vi "Configure Crop.vi"(8 "error in (no error)":errorcluster, 9 "Codec":string, 10 "Video file path":path, 11 "Frame Grabber Data In":T1={"Camera Session"="", "Frame"=refnum, "AVI Refnum"=refnum, "Codecs"=[], "Frame number"=0, "Tracking File Refnum"=refnum, "Tick Count"=0, "Probe Object"=refnum, "Playback Probe Data"=[], "Rigid Body"={"Position"={"x (mm)"=0.0, "y (mm)"=0.0, "z (mm)"=0.0}, "Orientation"={"Pitch (rad)"=0.0, "Yaw (rad)"=0.0, "Roll (rad)"=0.0}, "Quaternion"={"qx"=0.0, "qy"=0.0, "qz"=0.0, "qw"=0.0}, "Tracked?"=FALSE}, "Total no frames playback"=0, "Video FPS"=0.0, "Camera connected?"=FALSE, "Scene"=refnum, "Cropped Frame"=refnum, "Tracker FPS"=0.0, "Crop ROI"=[], "Presentation Values"=[], "Elapsed time (ms)"=0, "Camera frames playback"=0, "Refnums"={"Live Refnum"=refnum, "Record Refnum"=refnum, "Recording Settings Refnum"=refnum, "Playback Refnum"=refnum, "Frame Slider Refnum"=refnum, "Pause Refnum"=refnum, "Home Refnum"=refnum, "Crop Refnum"=refnum, "Clear Crop Refnum"=refnum, "stop refnum"=refnum, "Playback Rate Refnum"=refnum, "Operator Settings Refnums"=refnum, "Presentation Refnum"=refnum, "Gestation Refnum"=refnum, "Connection Settings Refnum"=refnum, "Crop Time Frame Slider Refnum"=refnum}, "Dimensions"={"Probe Dimensions"={"Probe Width"=0.0, "Probe Depth"=1.0, "Probe Height"=0.0}, "Room Dimensions"={"Room Width"=0.0, "Room Depth"=0.0, "Room Height"=0.0}}, "Playback Data As Strings"=[], "Cropped Tracking File Refnum"=refnum, "Cropped AVI Refnum"=refnum, "Header"=[]}) -> (0 "error out":errorcluster, 2 "Saving?":bool, 3 "Frame Grabber Data Out":T1={"Camera Session"="", "Frame"=refnum, "AVI Refnum"=refnum, "Codecs"=[], "Frame number"=0, "Tracking File Refnum"=refnum, "Tick Count"=0, "Probe Object"=refnum, "Playback Probe Data"=[], "Rigid Body"={"Position"={"x (mm)"=0.0, "y (mm)"=0.0, "z (mm)"=0.0}, "Orientation"={"Pitch (rad)"=0.0, "Yaw (rad)"=0.0, "Roll (rad)"=0.0}, "Quaternion"={"qx"=0.0, "qy"=0.0, "qz"=0.0, "qw"=0.0}, "Tracked?"=FALSE}, "Total no frames playback"=0, "Video FPS"=0.0, "Camera connected?"=FALSE, "Scene"=refnum, "Cropped Frame"=refnum, "Tracker FPS"=0.0, "Crop ROI"=[], "Presentation Values"=[], "Elapsed time (ms)"=0, "Camera frames playback"=0, "Refnums"={"Live Refnum"=refnum, "Record Refnum"=refnum, "Recording Settings Refnum"=refnum, "Playback Refnum"=refnum, "Frame Slider Refnum"=refnum, "Pause Refnum"=refnum, "Home Refnum"=refnum, "Crop Refnum"=refnum, "Clear Crop Refnum"=refnum, "stop refnum"=refnum, "Playback Rate Refnum"=refnum, "Operator Settings Refnums"=refnum, "Presentation Refnum"=refnum, "Gestation Refnum"=refnum, "Connection Settings Refnum"=refnum, "Crop Time Frame Slider Refnum"=refnum}, "Dimensions"={"Probe Dimensions"={"Probe Width"=0.0, "Probe Depth"=1.0, "Probe Height"=0.0}, "Room Dimensions"={"Room Width"=0.0, "Room Depth"=0.0, "Room Height"=0.0}}, "Playback Data As Strings"=[], "Cropped Tracking File Refnum"=refnum, "Cropped AVI Refnum"=refnum, "Header"=[]})   [LabVIEW 2017]
uses:
  Controls/Frame Grabber Data.ctl
  <vilib>/userdefined/High Color/IMAQdx.ctl
  <vilib>/vision/Image Controls.llb/IMAQ Image.ctl
  <vilib>/vision/Avi.llb/IMAQ AVI2 Refnum.ctl
  Controls/Rigid Body Info.ctl
  Controls/Position.ctl
  Controls/Orientation.ctl
  Controls/Refnums.ctl
  Controls/Recording Settings.ctl
  Controls/Operator Settings.ctl
  Controls/Operator.ctl
  Controls/Dimensions.ctl
  Controls/Room Dimensions.ctl
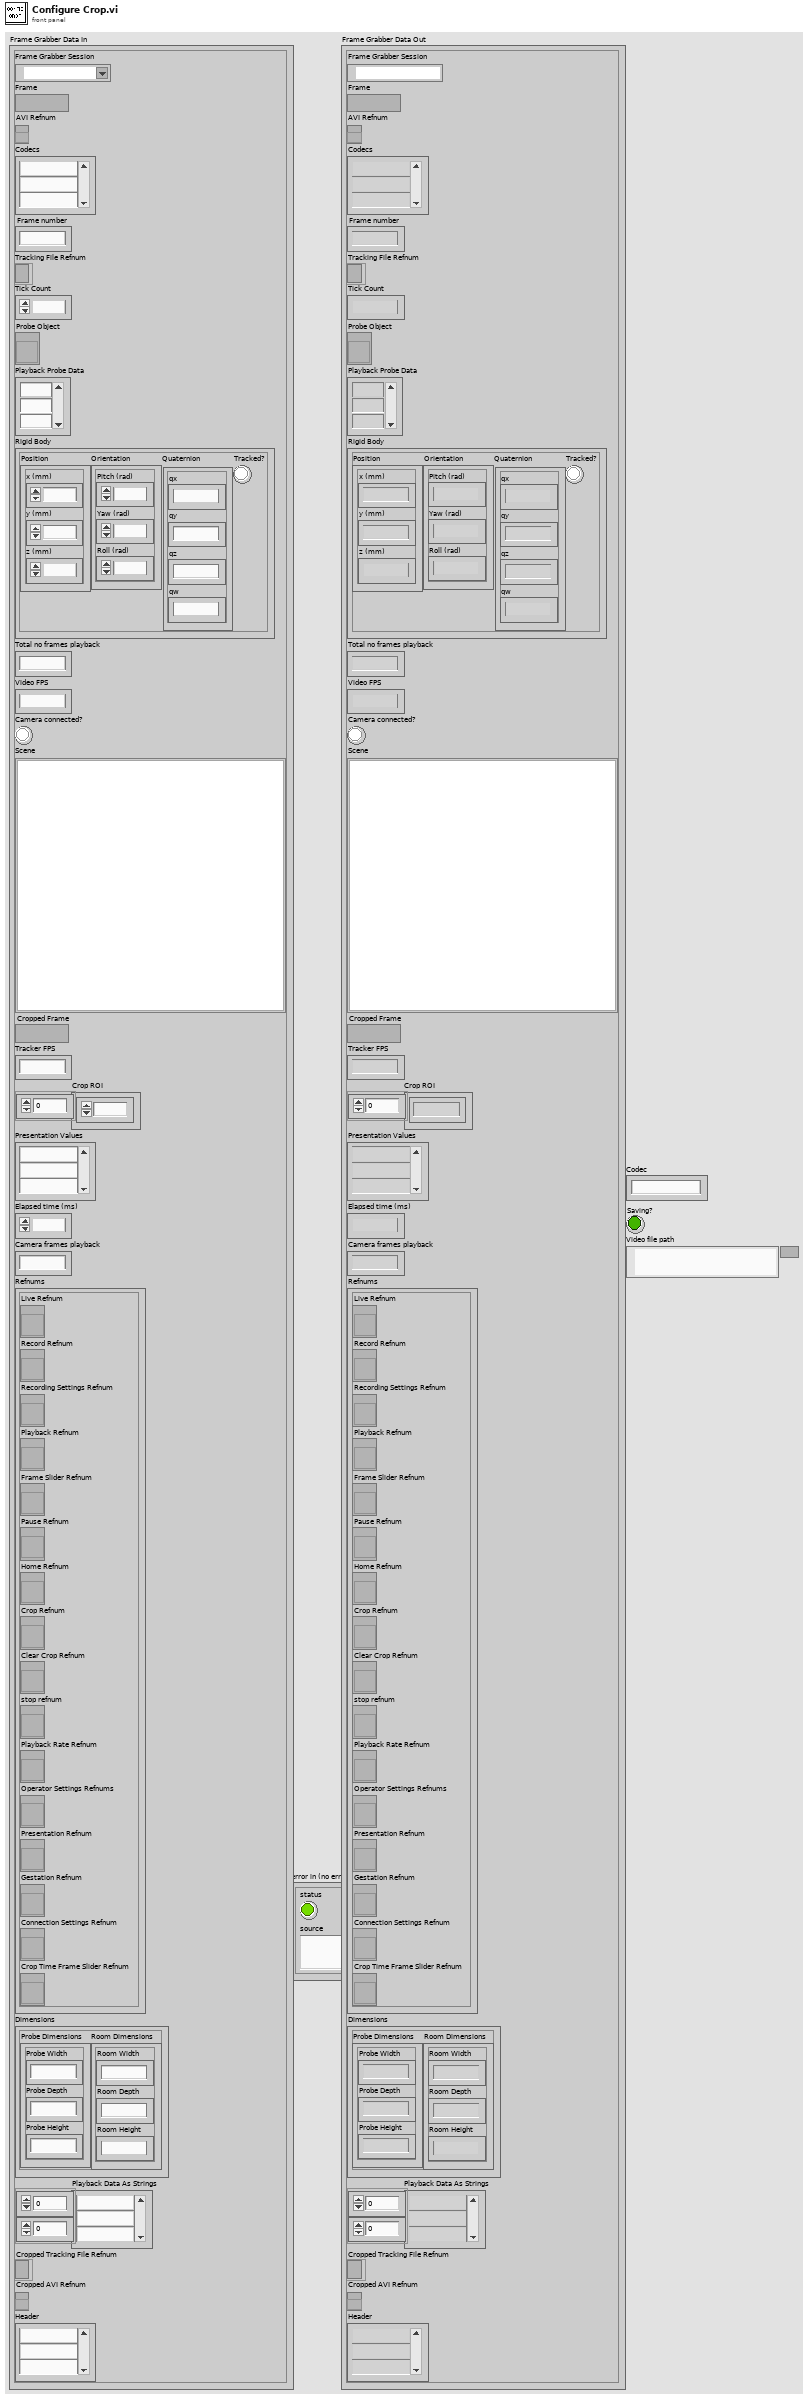
[diagram p1: front panel]
types:
  T1 = typedef "Frame Grabber Data.ctl" = cluster{"Camera Session":T2, "Frame":T3, "AVI Refnum":T4, "Codecs":string[], "Frame number":u32, "Tracking File Refnum":refnum<file>, "Tick Count":u32, "Probe Object":refnum<vi>, "Playback Probe Data":dbl[][], "Rigid Body":T5, "Total no frames playback":i32, "Video FPS":dbl, "Camera connected?":bool, "Scene":refnum<vi>, "Cropped Frame":T3, "Tracker FPS":dbl, "Crop ROI":i32[], "Presentation Values":string[], "Elapsed time (ms)":u32, "Camera frames playback":u32, "Refnums":T8, "Dimensions":T9, "Playback Data As Strings":string[][], "Cropped Tracking File Refnum":refnum<file>, "Cropped AVI Refnum":T4, "Header":string[]}
  T2 = typedef "IMAQdx.ctl" = refnum<k21>
  T3 = typedef "IMAQ Image.ctl" = refnum<image>
  T4 = typedef "IMAQ AVI2 Refnum.ctl" = refnum<k20>
  T5 = typedef "Rigid Body Info.ctl" = cluster{"Position":T6, "Orientation":T7, "Quaternion":cluster{"qx":sgl, "qy":sgl, "qz":sgl, "qw":sgl}, "Tracked?":bool}
  T6 = typedef "Position.ctl" = cluster{"x (mm)":sgl, "y (mm)":sgl, "z (mm)":sgl}
  T7 = typedef "Orientation.ctl" = cluster{"Pitch (rad)":sgl, "Yaw (rad)":sgl, "Roll (rad)":sgl}
  T8 = typedef "Refnums.ctl" = cluster{"Live Refnum":refnum<vi>, "Record Refnum":refnum<vi>, "Recording Settings Refnum":refnum<vi>, "Playback Refnum":refnum<vi>, "Frame Slider Refnum":refnum<vi>, "Pause Refnum":refnum<vi>, "Home Refnum":refnum<vi>, "Crop Refnum":refnum<vi>, "Clear Crop Refnum":refnum<vi>, "stop refnum":refnum<vi>, "Playback Rate Refnum":refnum<vi>, "Operator Settings Refnums":refnum<vi>, "Presentation Refnum":refnum<vi>, "Gestation Refnum":refnum<vi>, "Connection Settings Refnum":refnum<vi>, "Crop Time Frame Slider Refnum":refnum<vi>}
  T9 = typedef "Dimensions.ctl" = cluster{"Probe Dimensions":cluster{"Probe Width":sgl, "Probe Depth":sgl, "Probe Height":sgl}, "Room Dimensions":T10}
  T10 = typedef "Room Dimensions.ctl" = cluster{"Room Width":dbl, "Room Depth":dbl, "Room Height":dbl}
  T11 = enum16{"open", "replace", "create", "open or create", "replace or create", "replace or create with confirmation"}
  T12 = cluster{"Width":u32, "Height":u32, "Frames Per Second":u32, "Codec":string, "Has Data":bool}
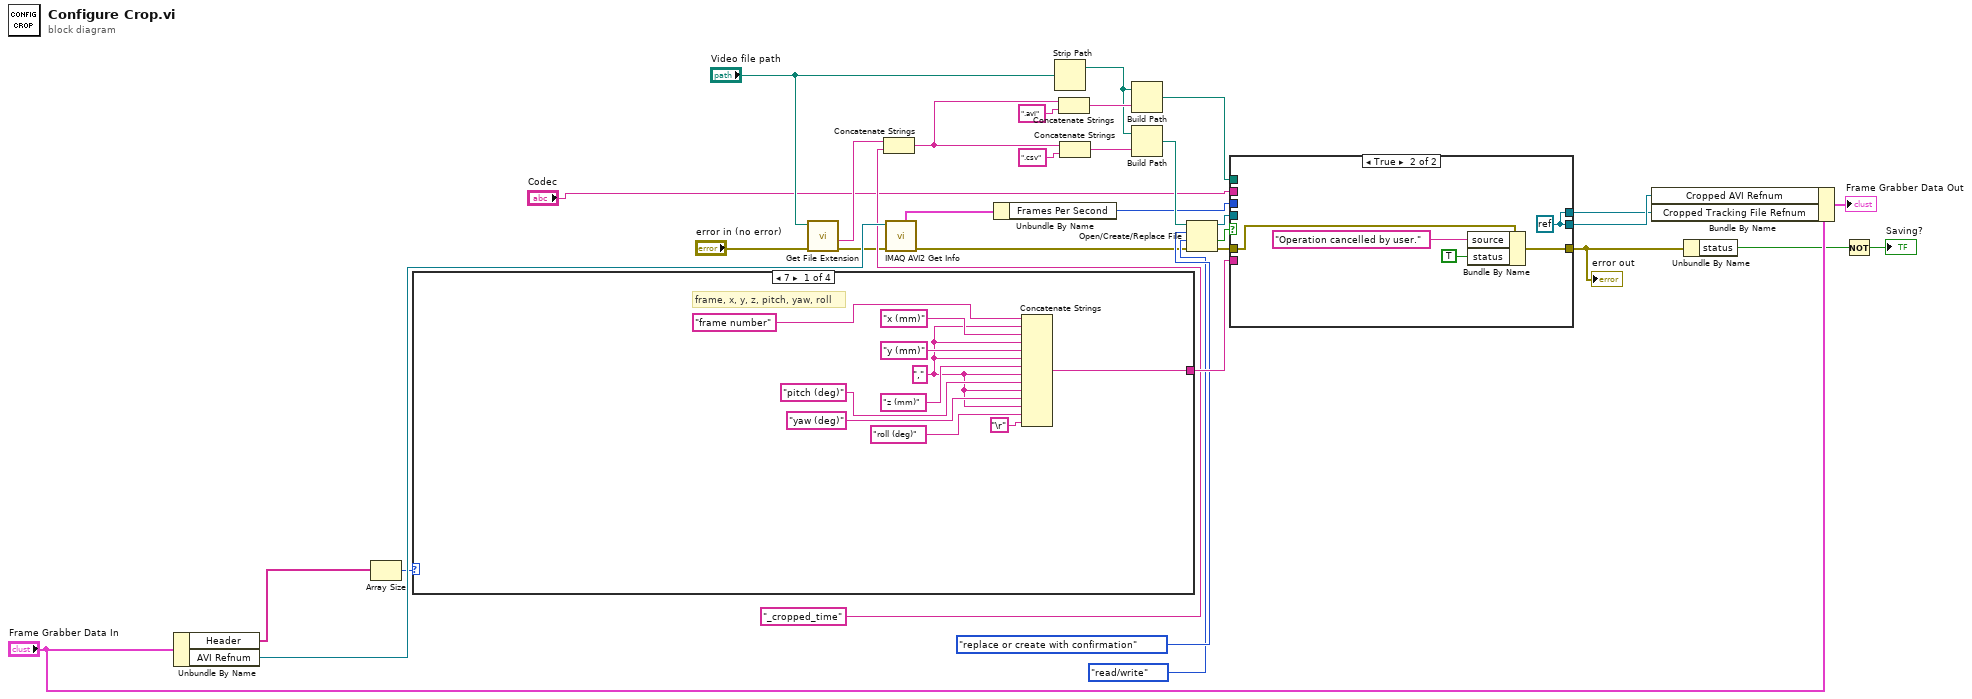
[diagram p0: block diagram]
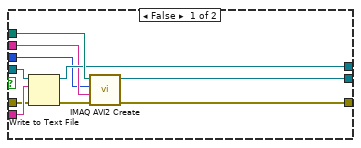
[diagram p2: hidden frame]
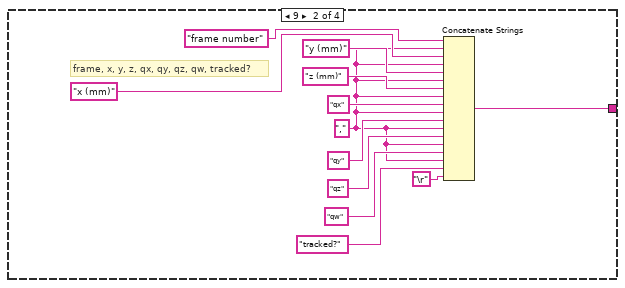
[diagram p3: hidden frame]
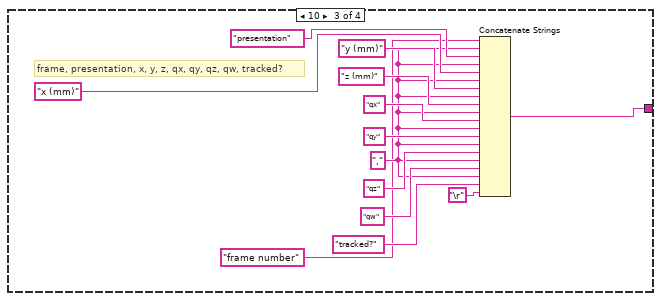
[diagram p4: hidden frame]
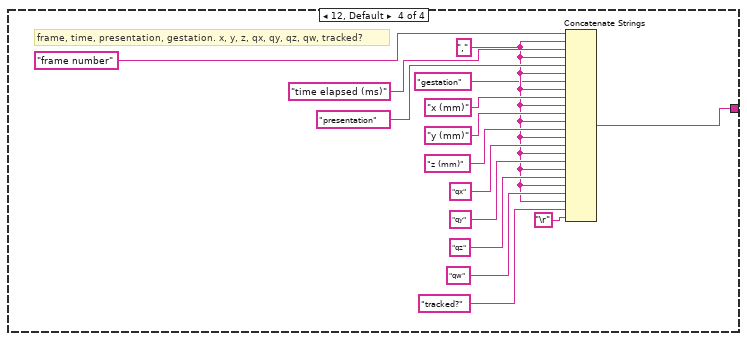
[diagram p5: hidden frame]
diagram:
  n1 = Unbundle By Name("Frame Grabber Data In") -> ("Header"=w2:string[], "AVI Refnum"=w16:T4)
  n2 = Array Size(array=w2) -> (size(s)=w8:i32)
  n3 = case shown="7" w8 {
    tunnel: [w35 w46 w56 w83] -> w33
    frame 7 {
      w34 = ","
      # "frame, x, y, z, pitch, yaw, roll"
      n4 = Concatenate Strings("frame number" ("string"), w34, "x (mm)" ("string"), w34, "y (mm)" ("string"), w34, "z (mm)" ("string"), w34, "pitch (deg)" ("string"), w34, "yaw (deg)" ("string"), w34, "roll (deg)" ("string"), "\r") -> (w35:string)
    }
    frame 9 {
      w47 = ","
      # "frame, x, y, z, qx, qy, qz, qw, tracked?"
      n5 = Concatenate Strings("frame number" ("string"), w47, "x (mm)" ("string"), w47, "y (mm)" ("string"), w47, "z (mm)" ("string"), w47, "qx" ("string"), w47, "qy" ("string"), w47, "qz" ("string"), w47, "qw" ("string"), w47, "tracked?" ("string"), "\r") -> (w46:string)
    }
    frame 10 {
      w58 = ","
      # "frame, presentation, x, y, z, qx, qy, qz, qw, tracked?"
      n6 = Concatenate Strings("frame number" ("string"), w58, "presentation" ("string"), w58, "x (mm)" ("string"), w58, "y (mm)" ("string"), w58, "z (mm)" ("string"), w58, "qx" ("string"), w58, "qy" ("string"), w58, "qz" ("string"), w58, "qw" ("string"), w58, "tracked?" ("string"), "\r") -> (w56:string)
    }
    frame 12, Default {
      w70 = ","
      # "frame, time, presentation, gestation. x, y, z, qx, qy, qz, qw, tracked?"
      n7 = Concatenate Strings("frame number" ("string"), w70, "time elapsed (ms)" ("string"), w70, "presentation" ("string"), w70, "gestation" ("string"), w70, "x (mm)" ("string"), w70, "y (mm)" ("string"), w70, "z (mm)" ("string"), w70, "qx" ("string"), w70, "qy" ("string"), w70, "qz" ("string"), w70, "qw" ("string"), w70, "tracked?" ("string"), "\r") -> (w83:string)
    }
  }
  n8 = call <vilib>:"Get File Extension.vi"("error in (no error)"="error in (no error)", "file"="Video file path") -> ("error out"=w9:errorcluster, "filename without extension"=w12:string)  [unwired: 5 in, 3 out]
  n9 = Concatenate Strings(w12, "_cropped_time" ("string")) -> (w6:string)
  n10 = call "IMAQ AVI2 Get Info"("error in (no error)"=w9, "AVI Refnum"=w16) -> ("error out"=w5:errorcluster, "Frame Data"=w15:T12)  [unwired: 5 in, 3 out]
  n11 = Unbundle By Name(w15) -> ("Frames Per Second"=w14:u32)
  n12 = Strip Path(path="Video file path") -> (stripped path=w7:path)  [unwired: 1 out]
  n13 = Concatenate Strings(w6, ".avi" ("string")) -> (w29:string)
  n14 = Concatenate Strings(w6, ".csv" ("string")) -> (w30:string)
  n15 = Build Path(base path=w7, name or relative path=w29) -> (appended path=w25:path)
  n16 = Build Path(base path=w7, name or relative path=w30) -> (appended path=w24:path)
  n17 = Open/Create/Replace File(file path (use dialog)=w24, error in=w5, operation (0:open)=T11."replace or create with confirmation", access (0:read/write)=enum16{"read/write", "read-only", "write-only"}."read/write") -> (refnum out=w22:refnum<file>, cancelled=w3:bool, error out=w23:errorcluster)  [unwired: 2 in]
  n18 = case shown="True" w3 {
    tunnel: w33 -> [w93 _]
    tunnel: [w92 w98] -> w27
    tunnel: w25 -> [w91 _]
    tunnel: w23 -> [w90 w97]
    tunnel: w22 -> [w89 _]
    tunnel: [w88 w98] -> w21
    tunnel: "Codec" -> [w87 _]
    tunnel: w14 -> [w86 _]
    tunnel: [w84 w96] -> w4
    frame False {
      n19 = Write to Text File(file (use dialog)=w89, text=w93, error in=w90) -> (refnum out=w88:refnum<file>, error out=w85:errorcluster)  [unwired: 1 in, 1 out]
      n20 = call "IMAQ AVI2 Create"("error in (no error)"=w85, "Codec"=w87, "Frames Per Second"=w86, "AVI Path"=w91) -> ("error out"=w84:errorcluster, "AVI Refnum"=w92:T4)  [unwired: 6 in]
    }
    frame True {
      w98 = refnum<k0> refnum
      n21 = Bundle By Name(cluster=w97, "source"="Operation cancelled by user.", "status"=TRUE) -> (w96:errorcluster)
    }
  }
  "error out" <- w4
  n22 = Bundle By Name(cluster="Frame Grabber Data In", "Cropped AVI Refnum"=w27, "Cropped Tracking File Refnum"=w21) -> (→"Frame Grabber Data Out":T1)
  n23 = Unbundle By Name(w4) -> ("status"=w18:bool)
  n24 = Not(x=w18) -> (.not. x?=→"Saving?":bool)
